vi "publish -- pll result.vi"(7 "publisher action":T2, 11 "pll result IN":T1={"freq (Hz)"=40017.438097734725, "gamma (Hz)"=0.0, "Voltage (V)"=6.817921124952451+0.0i, "overlimit ?"=FALSE} {"Voltage (V)" format="%#.4f"; "gamma (Hz)" format="%#.4f"; "freq (Hz)" format="%#.11f"}) -> (3 "pll result OUT":T1={"freq (Hz)"=40017.438097734725, "gamma (Hz)"=0.0, "Voltage (V)"=6.817921124952451+0.0i, "overlimit ?"=FALSE} {"Voltage (V)" format="%#.4f"; "gamma (Hz)" format="%#.4f"; "freq (Hz)" format="%#.11f"})   [LabVIEW 2018]
uses:
  pll talkback data type.ctl
  publisher action.ctl
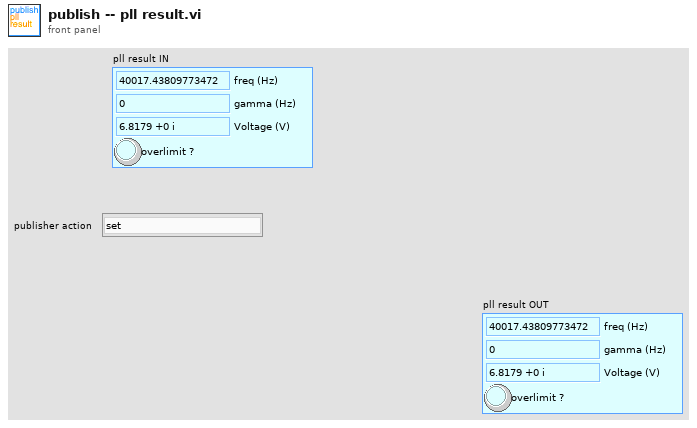
[diagram p1: front panel]
types:
  T1 = typedef "pll talkback data type.ctl" = cluster{"freq (Hz)":dbl, "gamma (Hz)":dbl, "Voltage (V)":cdb, "overlimit ?":bool}
  T2 = typedef "publisher action.ctl" = enum16{"set", "get", "init", "check"}
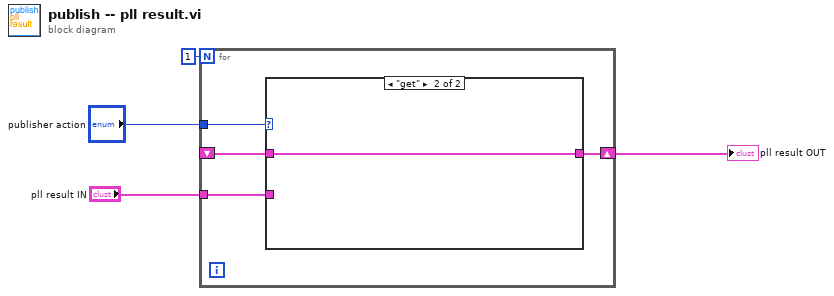
[diagram p0: block diagram]
diagram:
  n1 = for {
    N: 1 -> [_]
    tunnel: "publisher action" -> [w8]
    tunnel: "pll result IN" -> [w6]
    shift-right: [w7] -> w1
    shift-left: _ -> [w5]
    n2 = case shown="\"get\"" w8 {
      tunnel: [w9 w10] -> w7
      tunnel: w6 -> [w9 _]
      tunnel: w5 -> [_ w10]
      frame "set", Default {
      }
      frame "get" {
      }
    }
  }
  "pll result OUT" <- w1
